vi "Get Test Executive Version.vi"(7 "Unique ID":string, 8 "error in (no error)":errorcluster, 11 "Test Executive Ref":refnum<data-value>) -> (0 "error out":errorcluster, 1 "Found?":bool, 2 "Test Executive Version":string, 3 "Test Executive Ref out":refnum<data-value>)   [LabVIEW 2017, in "Test Executive.lvlib" / "TestExecutive Ref.lvclass"]
uses:
  <vilib>/gpm_packages/@cs/test-executive/Source/Test Executive/TestExecutive Ref/TestExecutive Ref.lvclass
  <vilib>/gpm_packages/@cs/test-executive/Source/Test Executive/ITestExecutive/ITest Executive.lvclass
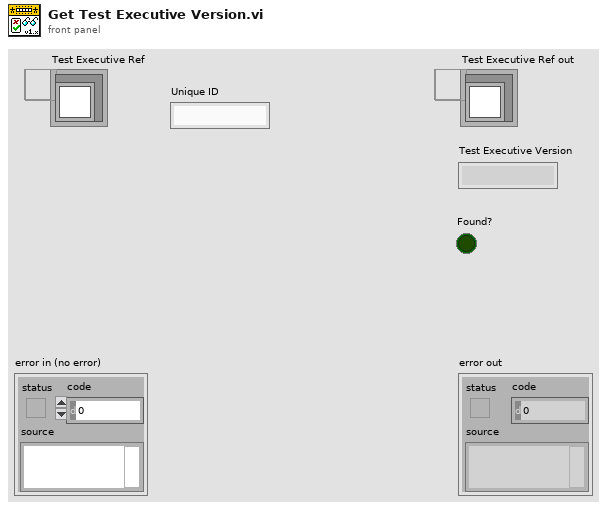
[diagram p1: front panel]
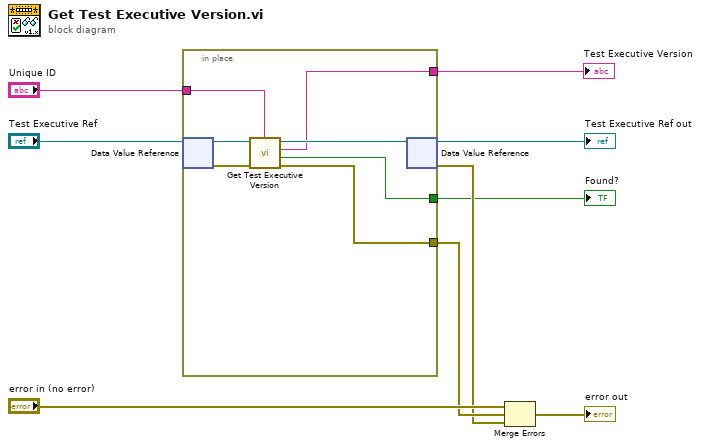
[diagram p0: block diagram]
diagram:
  n1 = in-place {
    in-place-border: "Unique ID" -> [w14]
    in-place-border: [w12] -> w5
    in-place-border: [w11] -> w2
    in-place-border: [w10] -> w1
    n2 = in-place-dvr #1("Test Executive Ref") -> (w16:refnum<class "ITest Executive.lvclass">, w13:errorcluster)
    n3 = call-dynamic "Get Test Executive Version.vi"("Unique ID"=w14, "error in (no error)"=w13, "ITest Executive in"=w16) -> ("error out"=w12:errorcluster, "Found?"=w10:bool, "Test Exec Version"=w11:string, "ITest Executive out"=w15:refnum<class "ITest Executive.lvclass">)  [unwired: 5 in]
    n4 = in-place-dvr #1(w15) -> (→"Test Executive Ref out":refnum<data-value>, w4:errorcluster)
  }
  "Test Executive Version" <- w2
  "Found?" <- w1
  n5 = Merge Errors("error in (no error)", w5, w4) -> (→"error out":errorcluster)
